vi "worker_loop.vi"(8 "error in (no error)":errorcluster, 10 "Notifiers":T1, 11 "Message Queues":T2) -> (0 "error out":errorcluster)   [LabVIEW 2017, in "worker.lvlib"]
uses:
  worker.lvlib
  support/Message Queue/All Message Queues.ctl
  support/Message Queue/Message Cluster.ctl
  support/Notifiers/Notifiers.ctl
  <vilib>/Utility/error.llb/Error Cluster From Error Code.vi
  <vilib>/ErrorRing/Error Ring.xnode
  support/Message Queue/Message Queue.lvlib
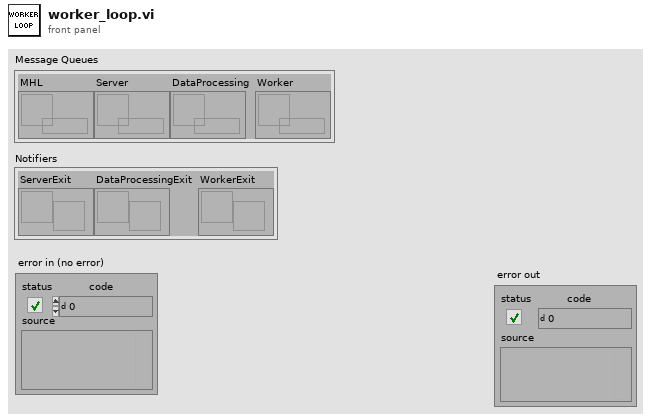
[diagram p1: front panel]
types:
  T1 = typedef "Notifiers.ctl" = cluster{"ServerExit":refnum<notifier>, "DataProcessingExit":refnum<notifier>, "WorkerExit":refnum<notifier>}
  T2 = typedef "Message Queue.lvlib/All Message Queues.ctl" = cluster{"MHL":refnum<queue>, "Server":refnum<queue>, "DataProcessing":refnum<queue>, "Worker":refnum<queue>}
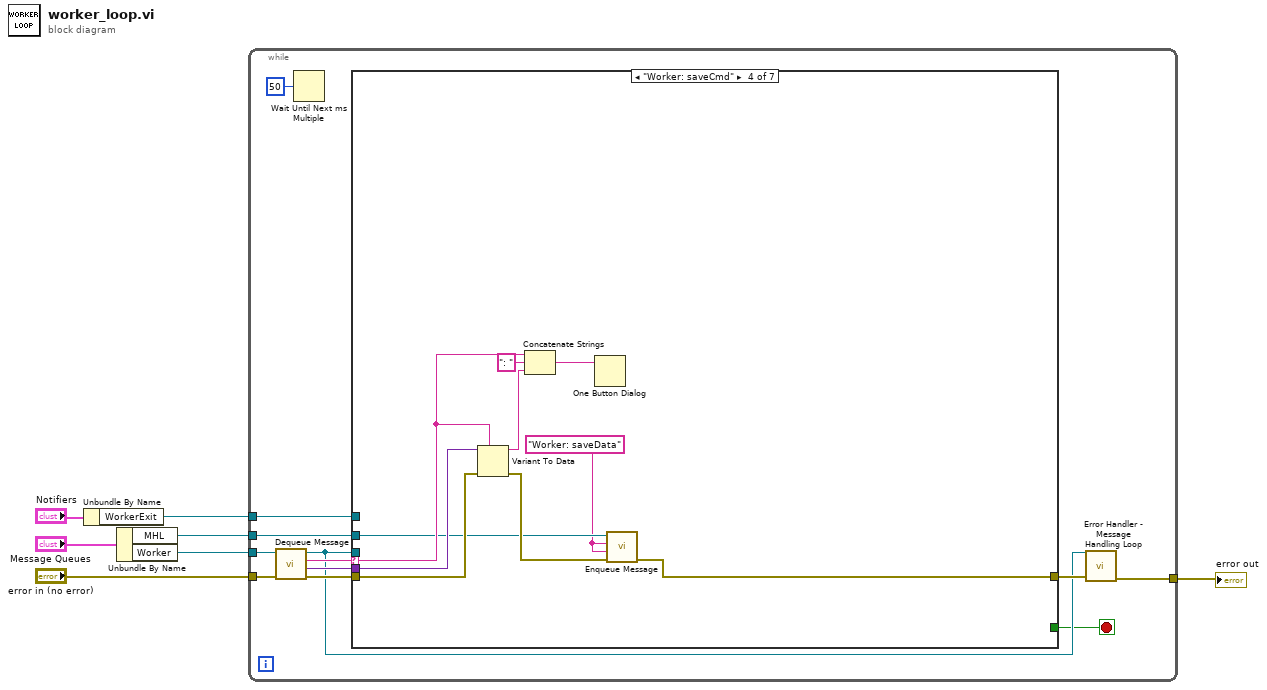
[diagram p0: block diagram]
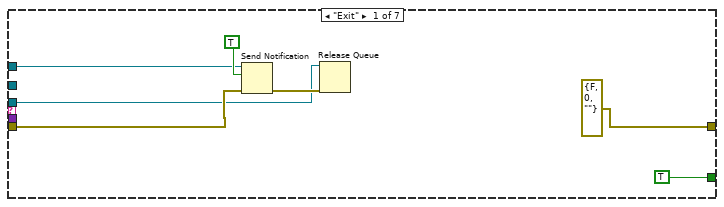
[diagram p2: hidden frame]
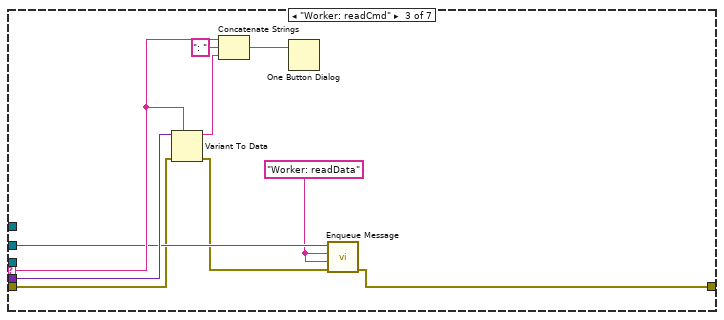
[diagram p4: hidden frame]
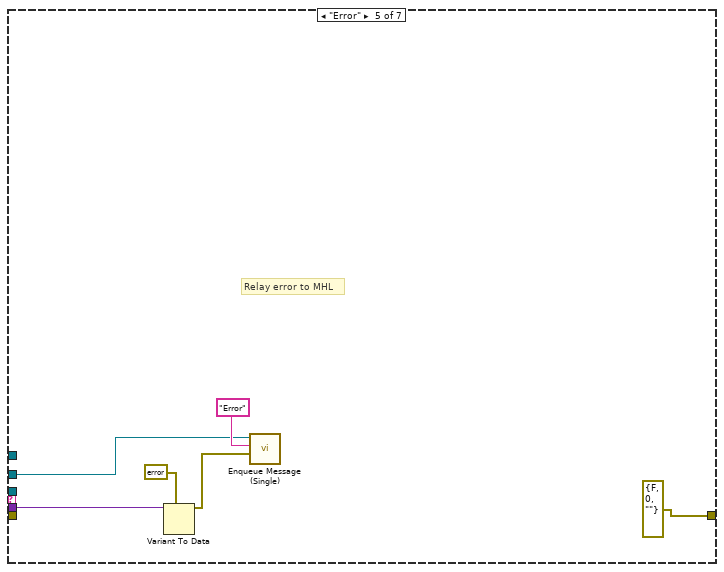
[diagram p5: hidden frame]
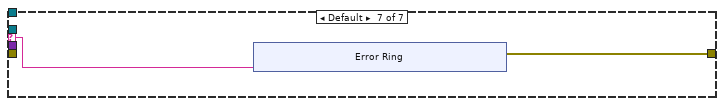
[diagram p7: hidden frame]
diagram:
  n1 = Unbundle By Name("Notifiers") -> ("WorkerExit"=w3:refnum<notifier>)
  n2 = Unbundle By Name("Message Queues") -> ("MHL"=w6:refnum<queue>, "Worker"=w5:refnum<queue>)
  n3 = while {
    tunnel: w6 -> [w13]
    tunnel: w5 -> [w18]
    tunnel: w3 -> [w8]
    tunnel: "error in (no error)" -> [w17]
    tunnel: [w10] -> w1
    stop <- w9 stop-if-true
    n4 = call "Dequeue Message.vi"("error in (no error)"=w17, "Message Queue"=w18) -> ("error out"=w14:errorcluster, "Message Data"=w15:variant, "Message"=w16:string, "dup Message Queue"=w11:refnum<queue>)  [unwired: 6 in]
    n5 = Wait Until Next ms Multiple(millisecond multiple=u32 50) -> ()  [unwired: 1 out]
    n6 = case shown="\"Worker: saveCmd\"" w16 {
      selector: w16 -> [_ _ w33 w44 _ _ w56]
      tunnel: w11 -> [w22 _ _ _ _ _ _]
      tunnel: w15 -> [_ _ w37 w45 w49 _ _]
      tunnel: w14 -> [w23 w27 w31 w41 _ w54 _]
      tunnel: w13 -> [_ _ w32 w39 w48 _ _]
      tunnel: [errorcluster {"status"=FALSE, "code"=0, "source"=""} ("error constant") w27 w29 w40 errorcluster {"status"=FALSE, "code"=0, "source"=""} ("error constant") w54 w55] -> w12
      tunnel: [TRUE _ _ _ _ _ _] -> w9
      tunnel: w8 -> [w21 _ _ _ _ _ _]
      frame "Exit" {
        n7 = Send Notification(notification=TRUE, notifier=w21, error in (no error)=w23) -> (error out=w24:errorcluster)  [unwired: 1 out]
        n8 = Release Queue(queue=w22, error in (no error)=w24) -> ()  [unwired: 1 in, 3 out]
      }
      frame "--- Copy me ---" {
      }
      frame "Worker: readCmd" {
        w28 = "Worker: readData" ("Message")
        n9 = Variant To Data(error in=w31, type=w33, Variant=w37) -> (data=w35:string, error out=w30:errorcluster)
        n10 = Concatenate Strings(w33, ": " ("string"), w35) -> (w34:string)
        n11 = One Button Dialog(message=w34) -> ()  [unwired: 1 in, 1 out]
        n12 = call-poly "Enqueue Message.vi"("error in (no error)"=w30, "Message Data"=w28, "Message"=w28, "Message Queue"=w32) -> ("error out"=w29:errorcluster)  [unwired: 6 in, 1 out]
      }
      frame "Worker: saveCmd" {
        w38 = "Worker: saveData" ("Message")
        n13 = Variant To Data(error in=w41, type=w44, Variant=w45) -> (data=w43:string, error out=w42:errorcluster)
        n14 = Concatenate Strings(w44, ": " ("string"), w43) -> (w46:string)
        n15 = One Button Dialog(message=w46) -> ()  [unwired: 1 in, 1 out]
        n16 = call-poly "Enqueue Message.vi"("error in (no error)"=w42, "Message Data"=w38, "Message"=w38, "Message Queue"=w39) -> ("error out"=w40:errorcluster)  [unwired: 6 in, 1 out]
      }
      frame "Error" {
        # "Relay error to MHL"
        n17 = Variant To Data(type=errorcluster {"status"=FALSE, "code"=0, "source"=""} ("error constant"), Variant=w49) -> (data=w51:errorcluster)  [unwired: 1 in, 1 out]
        n18 = call "Enqueue Message (Single).vi"("Message Data"=w51, "Message"="Error", "Message Queue"=w48) -> ()  [unwired: 7 in, 2 out]
      }
      frame "Initialize" {
      }
      frame Default {
        n19 = xnode "Error Ring"("parameter 0"=w56) -> ("error out"=w55:errorcluster)
      }
    }
    n20 = call "Error Handler - Message Handling Loop.vi"("error in (no error)"=w12, "Message Queue"=w11) -> ("dup error in"=w10:errorcluster)  [unwired: 8 in, 1 out]
  }
  "error out" <- w1
